vi "code_geneartiondaqmx.vi"() -> ()   [LabVIEW 2020]
uses:
  <vilib>/DAQmx/read.llb/DAQmx Read (Analog 1D Wfm NChan NSamp).vi
  <vilib>/DAQmx/miscellaneous.llb/DAQmx Fill In Error Info.vi
panel:
  out "data 2":dynamicdata(graph) caption="data"
  out "Sine":dynamicdata(graph)
  in  "stop":bool
  in  "stop (F)":bool
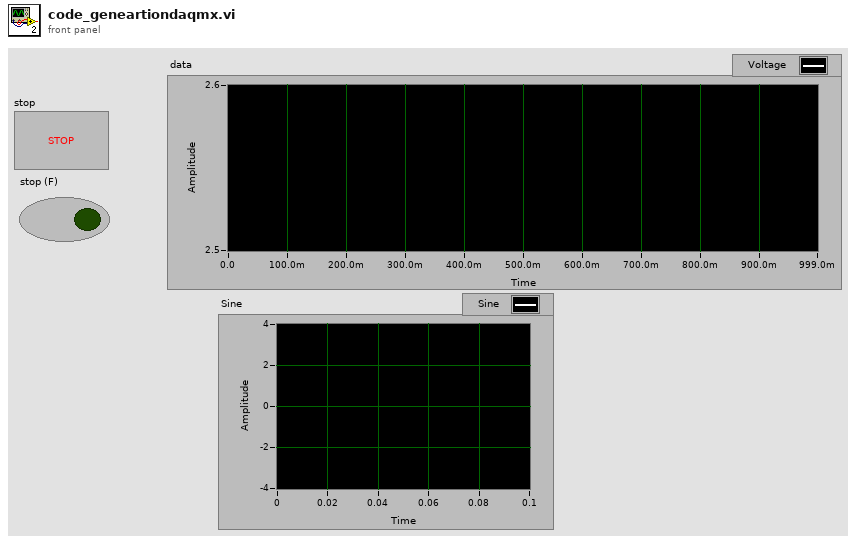
[diagram p1: front panel]
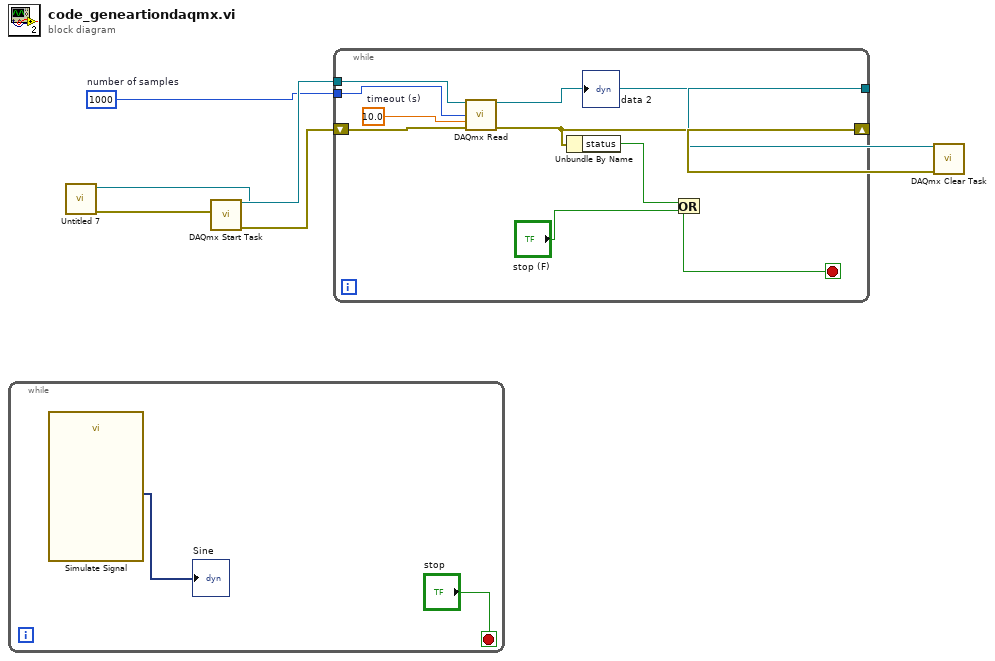
[diagram p0: block diagram]
diagram:
  w5 = 1000  # number of samples
  n1 = while {
    stop <- "stop" stop-if-true
    n2 = call "Simulate Signal"() -> ("Sine"=→"Sine":dynamicdata)  [unwired: 14 in, 1 out]
  }
  n3 = call "Untitled 7.vi"() -> ("error out"=w1:errorcluster, "task out"=w2:refnum<k21>)  [unwired: 10 in]
  n4 = call <vilib>:"DAQmx Start Task.vi"("task/channels in"=w2, "error in"=w1) -> ("task out"=w7:refnum<k21>, "error out"=w6:errorcluster)  [unwired: 12 in]
  n5 = while {
    tunnel: w7 -> [w18]
    tunnel: w5 -> [w15]
    tunnel: [w16] -> w3
    shift-right: [w13] -> w4
    shift-left: w6 -> [w17]
    stop <- w12 stop-if-true
    w11 = 10.0  # timeout (s)
    n6 = call-poly <vilib>:"DAQmx Read.vi"("task/channels in"=w18, "number of samples per channel"=w15, "timeout"=w11, "error in"=w17) -> ("task out"=w16:refnum<k21>, "error out"=w13:errorcluster)  [unwired: 9 in, 1 out]
    n7 = Unbundle By Name(w13) -> ("status"=w14:bool)
    n8 = Or(x=w14, y="stop (F)") -> (x .or. y?=w12:bool)
  }
  n9 = call <vilib>:"DAQmx Clear Task.vi"("task in"=w3, "error in"=w4) -> ()  [unwired: 13 in, 1 out]
